vi "Refresh_Map(SubVI).vi"(11 "Data Value Reference in":refnum<data-value>) -> ()   [LabVIEW 2017]
uses:
  <vilib>/robotics/Navigation/shared/WorldMap/OccupancyGridWorldMap/NI_Robotics_OccupancyGridWorldMap.lvclass
panel:
  out "error out":errorcluster
  in  "error in (no error)":errorcluster
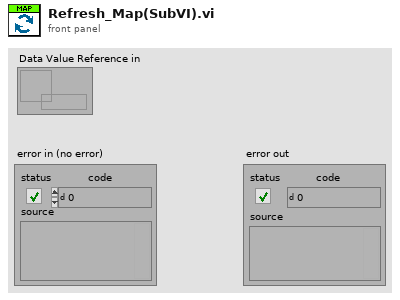
[diagram p1: front panel]
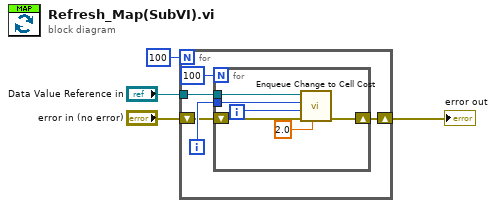
[diagram p0: block diagram]
diagram:
  n1 = for {
    N: 100 -> [_]
    tunnel: "Data Value Reference in" -> [w9]
    shift-right: [w6] -> w2
    shift-left: "error in (no error)" -> [w7]
    i -> [w8]
    n2 = for {
      N: 100 -> [_]
      tunnel: w9 -> [w15]
      tunnel: w8 -> [w14]
      shift-right: [w10] -> w6
      shift-left: w7 -> [w11]
      i -> [w13]
      n3 = call <vilib>:"Enqueue Change to Cell Cost.vi"("cost"=2.0, "error in (no error)"=w11, "y"=w13, "x"=w14, "map reference in"=w15) -> ("error out"=w10:errorcluster)  [unwired: 5 in, 1 out]
    }
  }
  "error out" <- w2
